vi "CRYSerial No.vi"(0 "Setup in":T1={"No.VI"=0, "Category"="", "StepName"="", "Seq setup flattened"="", "Comment"="", "Steps config."=[], "Jump config"=[], "Start"=0.0, "Increment"=0.0, "Name"="Pa", "Unit"="Pa", "Y data"=1, "Y prefix"="", "Y dB ref"=1.0, "Y unit"="", "Repeat State Array"=[]} {"Repeat State Array"."Start" format="%#_5g"; "Y dB ref" format="%.1f"; "Y data" items=["dB", "Lin"]; "Start" format="%#_5g"}, 5 "Data in":T4[](array[typedef]) {"Z data" items=["dB", "Lin"]; "X data" items=["dB", "Lin"]; "Y data" items=["dB", "Lin"]; "Z dB ref" format="%.1f"; "Z axis" items=["Log", "Lin"]; "X dB ref" format="%.1f"; "X axis" items=["Log", "Lin"]; "Y axis" items=["Log", "Lin"]; "Y dB ref" format="%.1f"; "Curve"."z" format="%.2f"; "Curve"."y" format="%.2f"; "Curve"."x" format="%.2f"}, 7 "Results in":T6 {"Margin" format="%.2f"}, 9 "Seq Setup in":string, 11 "Step name":string, 12 "Hardware in":string, 13 "Calibration in":string) -> (3 "Types Out":string[](array[string]), 4 "Inserted Names Out":string[](array[string]), 6 "Data Out":T4[](array[typedef]) {"Z data" items=["dB", "Lin"]; "X data" items=["dB", "Lin"]; "Y data" items=["dB", "Lin"]; "Z dB ref" format="%.1f"; "Z axis" items=["Log", "Lin"]; "X dB ref" format="%.1f"; "X axis" items=["Log", "Lin"]; "Y axis" items=["Log", "Lin"]; "Y dB ref" format="%.1f"; "Curve"."z" format="%.2f"; "Curve"."y" format="%.2f"; "Curve"."x" format="%.2f"}, 8 "Result Out":T5[](array[typedef]) {"Margin" format="%.2f"}, 10 "Waveform Out":T2 {"Y dB ref" format="%.1f"; "Y axis" items=["Log", "Lin"]; "Y data" items=["dB", "Lin"]; "X data" items=["dB", "Lin"]})   [LabVIEW 2013]
uses:
  Typedef Control/CRYData Cluster.ctl
  Typedef Control/CRYResult Cluster Array.ctl
  Typedef Control/CRYResult Cluster.ctl
  Typedef Control/CRYWaveform Cluster Array.ctl
  Typedef Control/CRYWaveform Cluster.ctl
  Typedef Control/CRYStep.ctl
  Data/CRYData & result stacks global.vi
  Task Sequence/CRYProject Run Control Global.vi
panel:
  in  "OK":bool
  in  "Serial Number":string
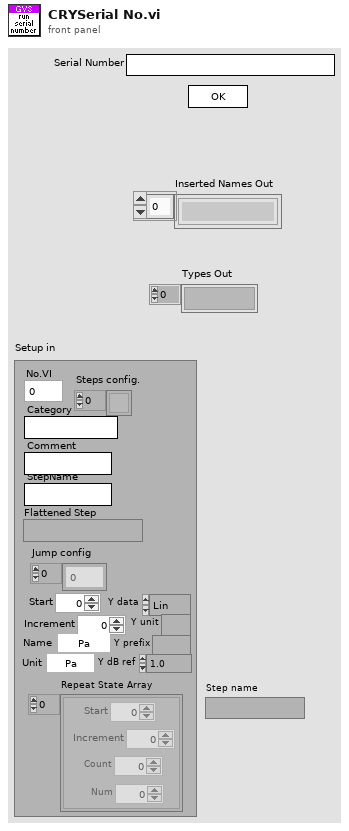
[diagram p1: front panel]
types:
  T1 = typedef "CRYStep.ctl" = cluster{"No.VI":i32, "Category":string, "StepName":string, "Seq setup flattened":string, "Comment":string, "Steps config.":bool[], "Jump config":i32[], "Start":dbl, "Increment":dbl, "Name":string, "Unit":string, "Y data":u16, "Y prefix":string, "Y dB ref":dbl, "Y unit":string, "Repeat State Array":cluster{"Start":dbl, "Increment":dbl, "Count":i32, "Num":i32}[]}
  T2 = typedef "CRYWaveform Cluster Array.ctl" = T3[]
  T3 = typedef "CRYWaveform Cluster.ctl" = cluster{"Waveform":cluster{"X0":dbl, "dX":dbl, "Y":sgl[]}, "X data":u16, "Y data":u16, "Y axis":u16, "X unit":string, "Y unit":string, "Y dB ref":dbl, "display Y":bool, "display X":bool, "Overload?":bool, "Test Info":string, "Step No.":i32, "Name":string, "protected":bool, "Sqc history":string[], "Signal Channel ID":i32, "Plot Settings":cluster{"Color":u32, "Interpolation":u8, "Point Style":u8, "Line Style":u8, "Point Color":u32, "Line Width":u8, "Bar Plot Style":u8, "Fill To":i16}, "AutoProtect":bool}
  T4 = typedef "CRYData Cluster.ctl" = cluster{"Name":string, "Curve":cluster{"x":dbl, "y":dbl, "z":dbl}[], "X data":u16, "Y data":u16, "Z data":u16, "X axis":u16, "Y axis":u16, "Z axis":u16, "X unit":string, "Y unit":string, "Z unit":string, "X dB ref":dbl, "Y dB ref":dbl, "Z dB ref":dbl, "single val":bool, "protected":bool, "display X":bool, "display Y":bool, "display Z":bool, "Test Info":string, "Step No.":i32, "Plot Settings":cluster{"Color":u32, "Interpolation":u8, "Point Style":u8, "Line Style":u8, "Point Color":u32, "Line Width":u8, "Bar Plot Style":u8, "Fill To":i16}, "AutoProtect":bool}
  T5 = typedef "CRYResult Cluster.ctl" = cluster{"Name":string, "Margin":dbl, "unit":string, "Verdict":bool, "Limit":string, "Max/Min":string, "protected":bool, "Step No.":i32, "Test Info":string, "AutoProtect":bool}
  T6 = typedef "CRYResult Cluster Array.ctl" = T5[]
  T7 = enum32{"Invalid", "Default", "Floating", "Floating/Auto-Hide", "Modal"}
  T8 = typedef "CRYSerial No.ctl" = cluster{"Name":string, "Mode":u16, "S/N prefix":string, "Tab Value":u16, "Help":string}
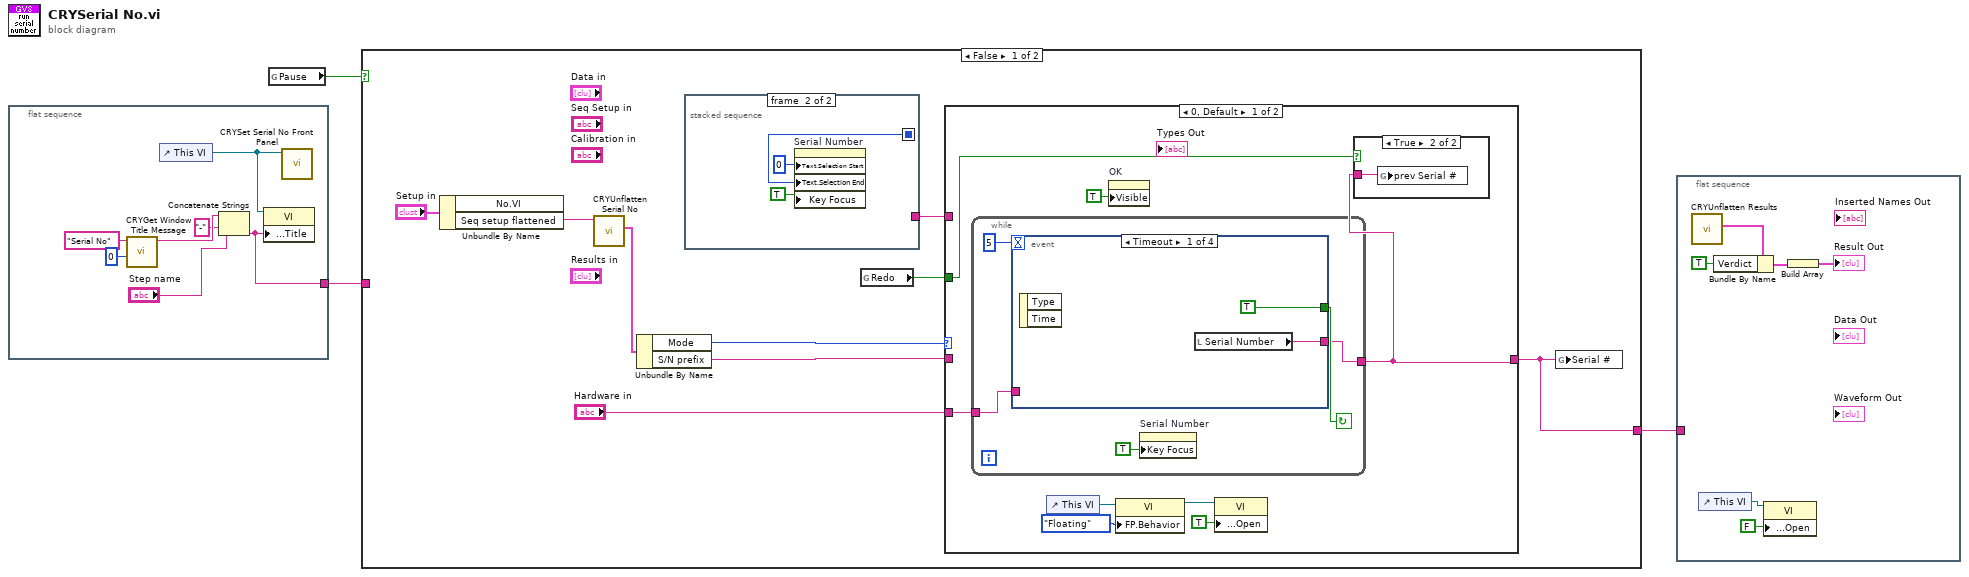
[diagram p0: block diagram]
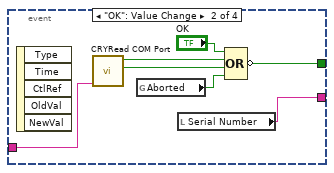
[diagram p3: hidden frame]
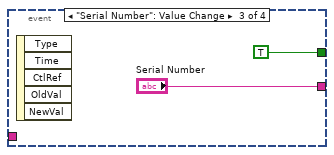
[diagram p4: hidden frame]
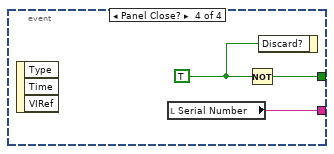
[diagram p5: hidden frame]
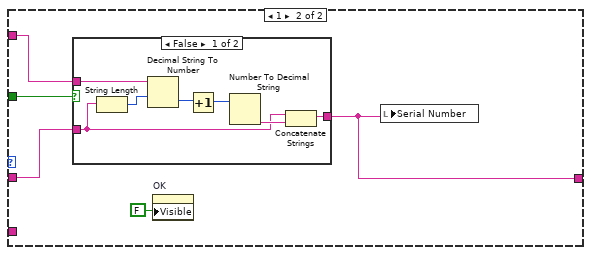
[diagram p6: hidden frame]
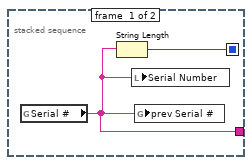
[diagram p8: hidden frame]
diagram:
  n1 = flat-sequence {
    tunnel: [w4] -> w1
    frame #0 {
      n2 = call "CRYGet Window Title Message.vi"("No"=0, "Kind"="Serial No") -> ("Multibyte String"=w8:string)  [unwired: 4 in, 5 out]
      n3 = control-ref of="This VI"() -> (w5:refnum<vi>)
      n4 = Concatenate Strings(w8, "-" ("string"), "Step name") -> (w4:string)
      n5 = property class="VI"(reference=w5, "Front Panel.Title"=w4) -> ()  [unwired: 1 in, 2 out]
      n6 = call "CRYSet Serial No Front Panel.vi"("Vi Ref"=w5) -> ()  [unwired: 11 in]
    }
  }
  n7 = global read "CRYData & result stacks global.vi" "Pause"() -> (w3:bool)
  n8 = case shown="False" w3 {
    tunnel: [w14 w66] -> w2
    tunnel: w1 -> [_ w66]
    frame False {
      n9 = Unbundle By Name("Setup in") -> ("Seq setup flattened"=w11:string)  [unwired: 1 out]
      n10 = call "CRYUnflatten Serial No.vi"("Unflatten Serial#"=w11) -> ("Serial#"=w13:T8)  [unwired: 8 in, 2 out]
      n11 = Unbundle By Name(w13) -> ("Mode"=w19:u16, "S/N prefix"=w16:string)
      n12 = stacked-sequence {
        seq-local: [w62 _] -> [_ w63]
        tunnel: [w61 _] -> w17
        frame #0 {
          n13 = global read "CRYData & result stacks global.vi" "Serial #"() -> (w61:string)
          n14 = String Length(string=w61) -> (length=w62:i32)
          n15 = local write "Serial Number"(w61) -> ()
          n16 = global write "CRYData & result stacks global.vi" "prev Serial #"(w61) -> ()
        }
        frame #1 {
          n17 = property on="Serial Number" class="Str"("Text.Selection Start"=u32 0 ("Text.Selection:Start"), "Text.Selection End"=w63, "Key Focus"=TRUE) -> ()  [unwired: 2 in, 2 out]
        }
      }
      n18 = global read "CRYData & result stacks global.vi" "Redo"() -> (w18:bool)
      n19 = case shown="0, Default" w19 {
        tunnel: w18 -> [w25 w51]
        tunnel: w17 -> [_ w50]
        tunnel: w16 -> [_ w49]
        tunnel: "Hardware in" -> [w26 _]
        tunnel: [w20 w48] -> w14
        frame 0, Default {
          n20 = while {
            tunnel: w26 -> [w33]
            tunnel: [w30] -> w20
            stop <- w31 continue-if-true
            n21 = event shown="[0] Timeout" {
              selector: _ -> [_ _ _ _]
              dyn-events: _ -> [_ _ _ _]
              timeout: 5 -> [_ _ _ _]
              tunnel: w33 -> [_ w38 _ _]
              tunnel: [TRUE w37 TRUE w46] -> w31
              tunnel: [w34 w36 "Serial Number" w45] -> w30
              event Timeout {
                n22 = event-data() -> ()  [unwired: 1 in, 2 out]
                n23 = local read "Serial Number"() -> (w34:string)
              }
              event "OK": Value Change {
                n24 = event-data() -> ()  [unwired: 1 in, 5 out]
                n25 = call "CRYRead COM Port.vi"("Hardware setup (if array not wired)"=w38) -> ("State 2 (Start & Continue)"=w41:bool, "State (Redo & Abort)"=w42:bool)  [unwired: 8 in, 1 out]
                n26 = global read "CRYProject Run Control Global.vi" "Aborted"() -> (w39:bool)
                n27 = local read "Serial Number"() -> (w36:string)
                n28 = Compound Arithmetic op=OR("OK", w42, w41, w39) -> (invert w37:bool)
              }
              event "Serial Number": Value Change {
                n29 = event-data() -> ()  [unwired: 1 in, 5 out]
              }
              event Panel Close? {
                w47 = TRUE ("Discard?")
                n30 = event-data() -> ()  [unwired: 1 in, 3 out]
                n31 = local read "Serial Number"() -> (w45:string)
                n32 = Not(x=w47) -> (.not. x?=w46:bool)
                n33 = event-data("Discard?"=w47) -> ()  [unwired: 1 in, 1 out]
              }
            }
            n34 = property on="Serial Number" class="Str"("Key Focus"=TRUE) -> ()  [unwired: 2 in, 2 out]
          }
          n35 = control-ref of="This VI"() -> (w22:refnum<vi>)
          n36 = property on="OK" class="Bool"("Visible"=TRUE) -> ()  [unwired: 2 in, 2 out]
          n37 = property class="VI"(reference=w22, "FP.Behavior"=T7."Floating" ("Front Panel Window:Behavior")) -> (reference out=w23:refnum<vi>)  [unwired: 1 in, 1 out]
          n38 = property class="VI"(reference=w23, "Front Panel.Open"=TRUE ("Front Panel Window:Open")) -> ()  [unwired: 1 in, 2 out]
          n39 = case shown="True" w25 {
            tunnel: w20 -> [_ w28]
            frame False {
            }
            frame True {
              n40 = global write "CRYData & result stacks global.vi" "prev Serial #"(w28) -> ()
            }
          }
        }
        frame 1 {
          n41 = case shown="False" w51 {
            tunnel: [w57 w60] -> w48
            tunnel: w49 -> [w55 _]
            tunnel: w50 -> [w53 w60]
            frame False {
              n42 = String Length(string=w55) -> (length=w54:i32)
              n43 = Decimal String To Number(string=w53, offset=w54) -> (number=w59:i32)  [unwired: 1 in, 1 out]
              n44 = Increment(x=w59) -> (x+1=w58:i32)
              n45 = Number To Decimal String(number=w58) -> (decimal integer string=w56:string)  [unwired: 1 in]
              n46 = Concatenate Strings(w55, w56) -> (w57:string)
            }
            frame True {
            }
          }
          n47 = property on="OK" class="Bool"("Visible"=FALSE) -> ()  [unwired: 2 in, 2 out]
          n48 = local write "Serial Number"(w48) -> ()
        }
      }
      n49 = global write "CRYData & result stacks global.vi" "Serial #"(w14) -> ()
    }
    frame True {
    }
  }
  n50 = flat-sequence {
    tunnel: w2 -> [_]
    frame #0 {
      n51 = call "CRYUnflatten Results.vi"() -> ("Result"=w68:T5)  [unwired: 9 in, 2 out]
      n52 = control-ref of="This VI"() -> (w67:refnum<vi>)
      n53 = Bundle By Name(cluster=w68, "Verdict"=TRUE) -> (w70:T5)
      n54 = property class="VI"(reference=w67, "Front Panel.Open"=FALSE ("Front Panel Window:Open")) -> ()  [unwired: 1 in, 2 out]
      n55 = Build Array(w70) -> (→"Result Out":T5[])
    }
  }
